vi "Clear CITI File.vi"(8 "error in (no error)":errorcluster, 11 "CITI reference in":refnum<k24>) -> (0 "error out":errorcluster, 3 "CITI reference out":refnum<k24>)   [LabVIEW 2023, in "NI_HFNetworkAnalysis.lvlib"]
doc: "Clear all CITI packages in memory for the referenced CITI file.\n\n<b>Note</b>\nThe actual content of the referenced CITI file on disk is not cleared."
uses:
  NI_HFNetworkAnalysis.lvlib
  C:/srd-semi-rfcal-software/AuxTools/STSRFFixtureCharactUtility/Source/Code Modules/Fixture/Dependencies/HFNetworkAnalysis/Support Files/NACE.Utils.Data.dll
  Support Files/NACE.Utils.Data.dll
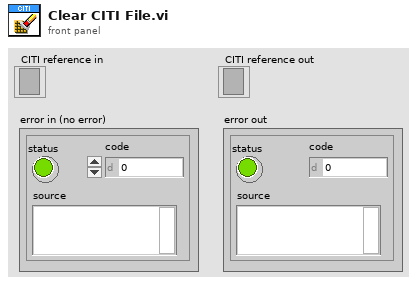
[diagram p1: front panel]
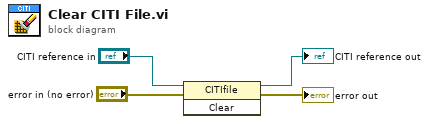
[diagram p0: block diagram]
diagram:
  n1 = invoke class="CITIfile" method="Clear"(reference="CITI reference in", error in="error in (no error)") -> (reference out=→"CITI reference out":refnum<k24>, error out=→"error out":errorcluster)  [unwired: 1 in, 1 out]
